vi "LidarRotateYZ.vi"(0 "Xin":i16, 1 "Theta_y (deg +/-250)":fxp<+/-,16,9>, 2 "Yin":i16, 3 "Zin":i16, 4 "Theta_z (deg +/-250)":fxp<+/-,16,9>) -> (5 "Xout":i16, 6 "Yout":i16, 7 "Zout":i16)   [LabVIEW 2010]
doc: "LidarRotateYZ.vi rotates a point in XYZ of LIDAR frame to XYZ in the gator's frame.\n\n<b>Inputs</b>\nXin - x position of point\nYin - y position of point\nZin - z position of point\nTheta_y - pitch of the LIDAR head in degrees below horizontal. Note that this only works for values in the range [-250,250].\nTheta_z - yaw of the LIDAR head in degrees left of forward. Note that this only works for values in the range [-250,250].\n\n<b>Outputs</b>\nXout - new x position of point\nYout - new y position of point\nZout - new z position of point"
uses:
  <vilib>/rvi/FXPMathLib/FxpSinAndCos/XNode/nifxpmath_SinAndCos.xnode
  <vilib>/rvi/FXPMathLib/FxpSinAndCos/subVIs/nifxpmath_SinAndCos_SimConfig.ctl
  <vilib>/rvi/FXPMathLib/FxpSinAndCos/simVIs/DllFxpSinAndCosTemp_sub.vi
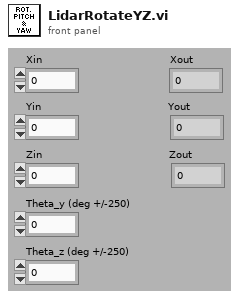
[diagram p1: front panel]
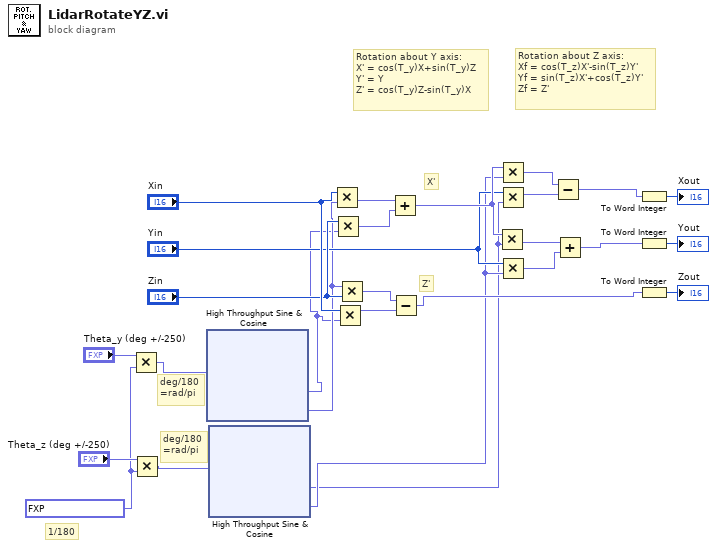
[diagram p0: block diagram]
diagram:
  w1 = fxp<+/-,16,0> 0.00555419921875
  # "deg/180\n=rad/pi"
  # "deg/180\n=rad/pi"
  # "1/180"
  # "Rotation about Z axis:\nXf = cos(T_z)X'-sin(T_z)Y'\nYf = sin(T_z)X'+cos(T_z)Y'\nZf = Z'"
  # "Rotation about Y axis:\nX' = cos(T_y)X+sin(T_y)Z\nY' = Y\nZ' = cos(T_y)Z-sin(T_y)X"
  # "Z'"
  # "X'"
  n1 = Multiply(x="Theta_y (deg +/-250)", y=w1) -> (x*y=w4:fxp<+/-,32,9>)
  n2 = Multiply(x="Theta_z (deg +/-250)", y=w1) -> (x*y=w2:fxp<+/-,32,9>)
  n3 = xnode "High Throughput Sine & Cosine"("x (pi)"=w4) -> ("sin(x)"=w8:fxp<+/-,16,2>, "cos(x)"=w9:fxp<+/-,16,2>)
  n4 = xnode "High Throughput Sine & Cosine"("x (pi)"=w2) -> ("sin(x)"=w6:fxp<+/-,16,2>, "cos(x)"=w7:fxp<+/-,16,2>)
  n5 = Multiply(x="Xin", y=w9) -> (x*y=w27:fxp<+/-,32,18>)
  n6 = Multiply(x="Zin", y=w8) -> (x*y=w26:fxp<+/-,32,18>)
  n7 = Multiply(x="Xin", y=w8) -> (x*y=w23:fxp<+/-,32,18>)
  n8 = Multiply(x=w9, y="Zin") -> (x*y=w25:fxp<+/-,32,18>)
  n9 = Add(x=w27, y=w26) -> (x+y=w11:fxp<+/-,33,19>)
  n10 = Subtract(x=w25, y=w23) -> (x-y=w18:fxp<+/-,32,18>)
  n11 = Multiply(x=w11, y=w6) -> (x*y=w14:fxp<+/-,47,19>)
  n12 = Multiply(x=w11, y=w7) -> (x*y=w16:fxp<+/-,47,19>)
  n13 = Multiply(x="Yin", y=w6) -> (x*y=w17:fxp<+/-,32,18>)
  n14 = Multiply(x="Yin", y=w7) -> (x*y=w15:fxp<+/-,32,18>)
  n15 = Subtract(x=w16, y=w17) -> (x-y=w12:fxp<+/-,48,20>)
  n16 = Add(x=w14, y=w15) -> (x+y=w13:fxp<+/-,48,20>)
  n17 = To Word Integer(number=w12) -> (16bit integer=→"Xout":i16)
  n18 = To Word Integer(number=w13) -> (16bit integer=→"Yout":i16)
  n19 = To Word Integer(number=w18) -> (16bit integer=→"Zout":i16)
